vi "Close.vi"(8 "error in":errorcluster, 11 "Humidity Actual Value in":refnum<class "Humidity Actual Value.lvclass">) -> (0 "error out":errorcluster, 3 "Humidity Actual Value out":refnum<class "Humidity Actual Value.lvclass">)   [LabVIEW 2023, in "Humidity Actual Value.lvclass"]
uses:
  Humidity Actual Value.lvclass
  Humidity Actual Value.lvclass/Humidity Actual Value.ctl
  Parents/Actual Value/Actual Value.lvclass
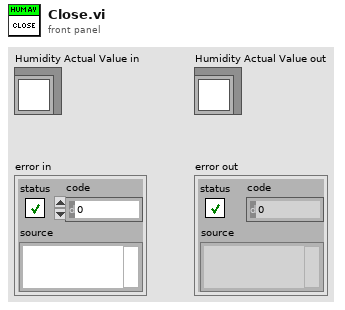
[diagram p1: front panel]
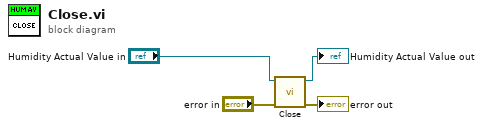
[diagram p0: block diagram]
diagram:
  n1 = call-parent "Close.vi"("error in"="error in", "Actual Value in"="Humidity Actual Value in") -> ("error out"=→"error out":errorcluster, "Actual Value out"=→"Humidity Actual Value out":refnum<class "Humidity Actual Value.lvclass">)  [unwired: 8 in]
